vi "_systemErrorClusterReplacement.vi"(8 "error in (no error)":errorcluster, 11 "Folder Path":path) -> (0 "error out":errorcluster)   [LabVIEW 2017]
doc: "Replaces current Error cluster (in and out) by the System Error Cluster."
uses:
  <vilib>/Utility/traverseref.llb/TRef TravTarget.ctl
panel:
  out "progress":string
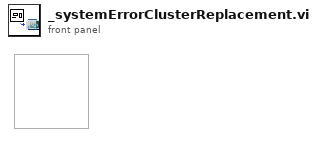
[diagram p1: front panel]
types:
  T1 = enum32{"Invalid", "Standard", "Closed", "Hidden", "Minimized", "Maximized"}
  T2 = typedef "TRef TravTarget.ctl" = enum16{"FP", "BD", "Other"}
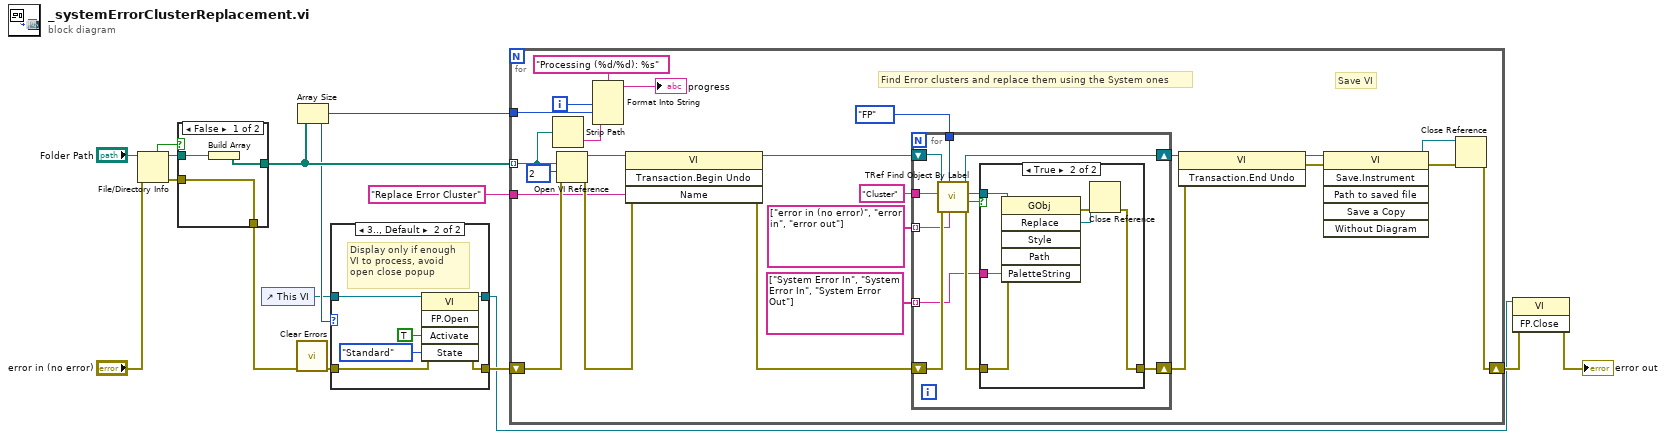
[diagram p0: block diagram]
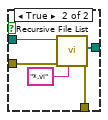
[diagram p2: hidden frame]
diagram:
  n1 = File/Directory Info(path="Folder Path", error in="error in (no error)") -> (path out=w9:path, directory=w7:bool, error out=w8:errorcluster)  [unwired: 4 out]
  n2 = case shown="False" w7 {
    tunnel: [w16 w22] -> w15
    tunnel: [w17 w21] -> w14
    tunnel: w9 -> [w18 w20]
    tunnel: w8 -> [w17 w19]
    frame False {
      n3 = Build Array(w18) -> (w16:path[])
    }
    frame True {
      n4 = call <vilib>:"Recursive File List.vi"("pattern"="*.vi", "error in (no error)"=w19, "Folder Path"=w20) -> ("error out"=w21:errorcluster, "All Files in Dir"=w22:path[])  [unwired: 4 in, 3 out]
    }
  }
  n5 = control-ref of="This VI"() -> (w1:refnum<vi>)
  n6 = call <vilib>:"Clear Errors.vi"("error in (no error)"=w14) -> ("error out"=w2:errorcluster)  [unwired: 5 in, 1 out]
  n7 = Array Size(array=w15) -> (size(s)=w3:i32)
  n8 = case shown="3.., Default" w3 {
    tunnel: w2 -> [w25 w29]
    tunnel: [w25 w28] -> w13
    tunnel: w1 -> [w24 w27]
    tunnel: [w24 w26] -> w4
    frame 0..2 {
    }
    frame 3.., Default {
      # "Display only if enough\nVI to process, avoid \nopen close popup"
      n9 = invoke class="VI" method="FP.Open"(reference=w27, error in=w29, "Activate"=TRUE ("Activate?"), "State"=T1."Standard") -> (reference out=w26:refnum<vi>, error out=w28:errorcluster)  [unwired: 1 in, 3 out]
    }
  }
  n10 = for {
    shift-right: [w48] -> w12
    shift-left: w13 -> [w46]
    tunnel: w15 -> [w44] mode=indexing
    tunnel: w3 -> [w41]
    tunnel: "Replace Error Cluster" ("Name") -> [w35]
    i -> [w43]
    # "Save VI"
    # "Find Error clusters and replace them using the System ones"
    n11 = Strip Path(path=w44) -> (name=w40:string)  [unwired: 1 out]
    n12 = Open VI Reference(vi path=w44, options=2, error in (no error)=w46) -> (vi reference=w47:refnum<vi>, error out=w37:errorcluster)  [unwired: 3 in]
    n13 = Format Into String(format string="Processing (%d/%d): %s", w43, w41, w40) -> (resulting string=→"progress":string)  [unwired: 2 in, 1 out]
    n14 = invoke class="VI" method="Transaction.Begin Undo"(reference=w47, error in=w37, "Name"=w35) -> (reference out=w38:refnum<vi>, error out=w36:errorcluster)  [unwired: 1 in, 2 out]
    n15 = for {
      tunnel: TRef_TravTarget."FP" ("Traverse Target") -> [w65]
      tunnel: "Cluster" ("Class Name") -> [w64]
      shift-right: [w61] -> w51
      shift-left: w38 -> [w66]
      tunnel: string[] ["error in (no error)", "error in", "error out"] -> [w57] mode=indexing
      tunnel: string[] ["System Error In", "System Error In", "System Error Out"] -> [w56] mode=indexing
      shift-right: [w60] -> w50
      shift-left: w36 -> [w58]
      n16 = call <vilib>:"TRef Find Object By Label.vi"("Label"=w57, "Traverse Target"=w65, "error in (no error)"=w58, "Class Name"=w64, "VI Ref"=w66) -> ("error out"=w62:errorcluster, "Found?"=w59:bool, "Found Obj Ref"=w63:refnum<vi>, "dup VI Ref"=w61:refnum<vi>)  [unwired: 3 in]
      n17 = case shown="True" w59 {
        tunnel: w63 -> [_ w73]
        tunnel: w62 -> [w67 w72]
        tunnel: w56 -> [_ w71]
        tunnel: [w67 w69] -> w60
        frame False {
        }
        frame True {
          n18 = invoke class="GObj" method="Replace"(reference=w73, error in=w72, "PaletteString"=w71) -> (error out=w70:errorcluster, "Replace"=w68:refnum<vi>)  [unwired: 3 in, 4 out]
          n19 = Close Reference(reference=w68, error in (no error)=w70) -> (error out=w69:errorcluster)
        }
      }
    }
    n20 = invoke class="VI" method="Transaction.End Undo"(reference=w51, error in=w50) -> (reference out=w49:refnum<vi>, error out=w32:errorcluster)  [unwired: 1 in, 1 out]
    n21 = invoke class="VI" method="Save.Instrument"(reference=w49, error in=w32) -> (reference out=w34:refnum<vi>, error out=w33:errorcluster)  [unwired: 4 in, 4 out]
    n22 = Close Reference(reference=w34, error in (no error)=w33) -> (error out=w48:errorcluster)
  }
  n23 = invoke class="VI" method="FP.Close"(reference=w4, error in=w12) -> (error out=→"error out":errorcluster)  [unwired: 1 in, 2 out]
